vi "Sync clocks.vi"() -> ()   [LabVIEW 2019]
uses:
  <vilib>/Utility/error.llb/DialogType.ctl
  <vilib>/DAQmx/write.llb/DAQmx Write (Analog 2D DBL NChan NSamp).vi
  <vilib>/DAQmx/read.llb/DAQmx Read (Analog 2D DBL NChan NSamp).vi
  <vilib>/DAQmx/create/channels.llb/DAQmx Create Channel (AI-Voltage-Basic).vi
  <vilib>/DAQmx/configure/timing.llb/DAQmx Timing (Sample Clock).vi
  <vilib>/DAQmx/configure/trigger.llb/DAQmx Reference Trigger (Digital Edge).vi
  <vilib>/DAQmx/create/channels.llb/DAQmx Create Channel (AO-Voltage-Basic).vi
  <vilib>/DAQmx/configure/trigger.llb/DAQmx Start Trigger (Digital Edge).vi
  <vilib>/DAQmx/configure/trigger.llb/DAQmx Start Trigger (Time).vi
  <vilib>/DAQmx/configure/trigger.llb/DAQmx Start Trigger (Analog Edge).vi
  <vilib>/DAQmx/miscellaneous.llb/DAQmx Fill In Error Info.vi
  <resource>/objmgr/daqmx.rc
panel:
  out "standard output":string
  out "standard error":string
  out "return code":i32
  out "error out":errorcluster
  in  "command line":string
  in  "standard input":string
  in  "error in (no error)":errorcluster
  out "Execution Time (ms)":u32=13382
  out "Stop Tick":u32=2219165183
  out "Start Tick":u32=2219151801
  out "Acquired Samples":dbl[][](array[numeric]) format="%0.2f"
  out "Acquired Data":dbl[][](graph)
  out "Sampled Data Array Size":i32[](array[numeric])
  out "number of samples written per channel":u32
  out "binaryArraySize":i32[](array[numeric])
  in  "Transmit File Path":path=path "/media/sdc1/TempOATS1.bin"
  out "Current Acquired Data File":path=path "/media/sdc1/Temp220825212226.bin"
  in  "File Name Prefix":string="Temp"
  in  "path 2":path=path "/media/sdc1"
  out "free (bytes)":i64=2925575569408
  out "size (bytes)":i64=2999825367040
  out "folder names":string[](array[string])=["$RECYCLE.BIN", "29_Mar_noWind_Wave", "30_Mar_pier", "31_Mar_pier", "Bootcamp_recordings_SOARS", "IMTLab Wave Maker-12-21-21", "SOARS Software IMT Lab 032422", "System Volume Information", "TFOBootcamp2022_Day2", "TFO_Day3_signals", "TFO_Day4_signals", "temp"]
  out "filenames":string[](array[string])=[".dropbox.device", "Crack open SOARS binary log file 032422.vi", "IMTLab SOARS Datalogger.vi", "PolarPulldown_032422.bin", "Temp.bin", "Temp220407000420.bin", "Temp220825212058.bin", "Temp220825212226.bin"]
  in  "cDAQ Data File Path":path=path "/media/sdc1"
  in  "AI pretrigger samples per channel":u32=2
  in  "AI Trigger Edge":i32(ring)=10280 items=["Rising"=10280, "Falling"=10171]
  in  "AI Trigger Source":tag="/cDAQ1/ao/SampleClock"
  out "AI SampClk.Rate":dbl
  in  "AI Clock Source":tag="OnboardClock"
  in  "physical channels":tag="cDAQ1Mod1/ai0:3"
  in  "Trigger Type":T1(tab)
  in  "Digital Start Trigger Edge":i32(ring)=10280 caption="Edge" items=["Rising"=10280, "Falling"=10171]
  in  "Digital Start Trigger Source":tag="/Dev1/PFI0" caption="Source"
  in  "Digital Pause Trigger Pause When":i32(ring)=10192 caption="Pause When" items=["High"=10192, "Low"=10214]
  in  "Digital Pause Trigger Source":tag="/Dev1/PFI0" caption="Source"
  in  "Analog Start Trigger Level":dbl caption="Level" format="%0.2f"
  in  "Analog Start Trigger Hysteresis":dbl caption="Hysteresis" format="%.2f"
  in  "Analog Start Trigger Slope":i32(ring)=10280 caption="Slope" items=["Rising"=10280, "Falling"=10171]
  in  "Analog Start Trigger Source":string="APFI0" caption="Source"
  in  "Analog Pause Trigger Source":string="APFI0" caption="Source"
  in  "Analog Pause Trigger Pause When":i32(ring)=10093 caption="Pause When" items=["Above Level"=10093, "Below Level"=10107]
  in  "Analog Pause Trigger Level":dbl caption="Level" format="%.2f"
  in  "When":timestamp
  in  "Select Time\nManually":bool
  out "Data to Transmit":dbl[][](graph)
  out "Number of Samples":i32
  in  "Sample Rate":dbl=1000000.0
  in  "AO Sample Clock Source":tag="OnboardClock"
  in  "Max Voltage":dbl=5.0
  in  "Min Voltage":dbl=-5.0
  in  "Physical Channel(s)":tag="cDAQ1Mod2/ao0:3"
  out "Actual Sample Rate":dbl format="%0.2f"
  # "To enable triggers, select a tab above, and configure the settings.\n\nNot all hardware supports all trigger types. Refer to your device documentation for more information."
  # "This trigger type is not supported in output tasks. \n\nRefer to your device documentation for more information on which triggers are supported."
  # "This trigger type is not supported in output tasks. \n\nRefer to your device documentation for more information on which triggers are supported."
  # "If time is not manually set, task will begin after 10 seconds"
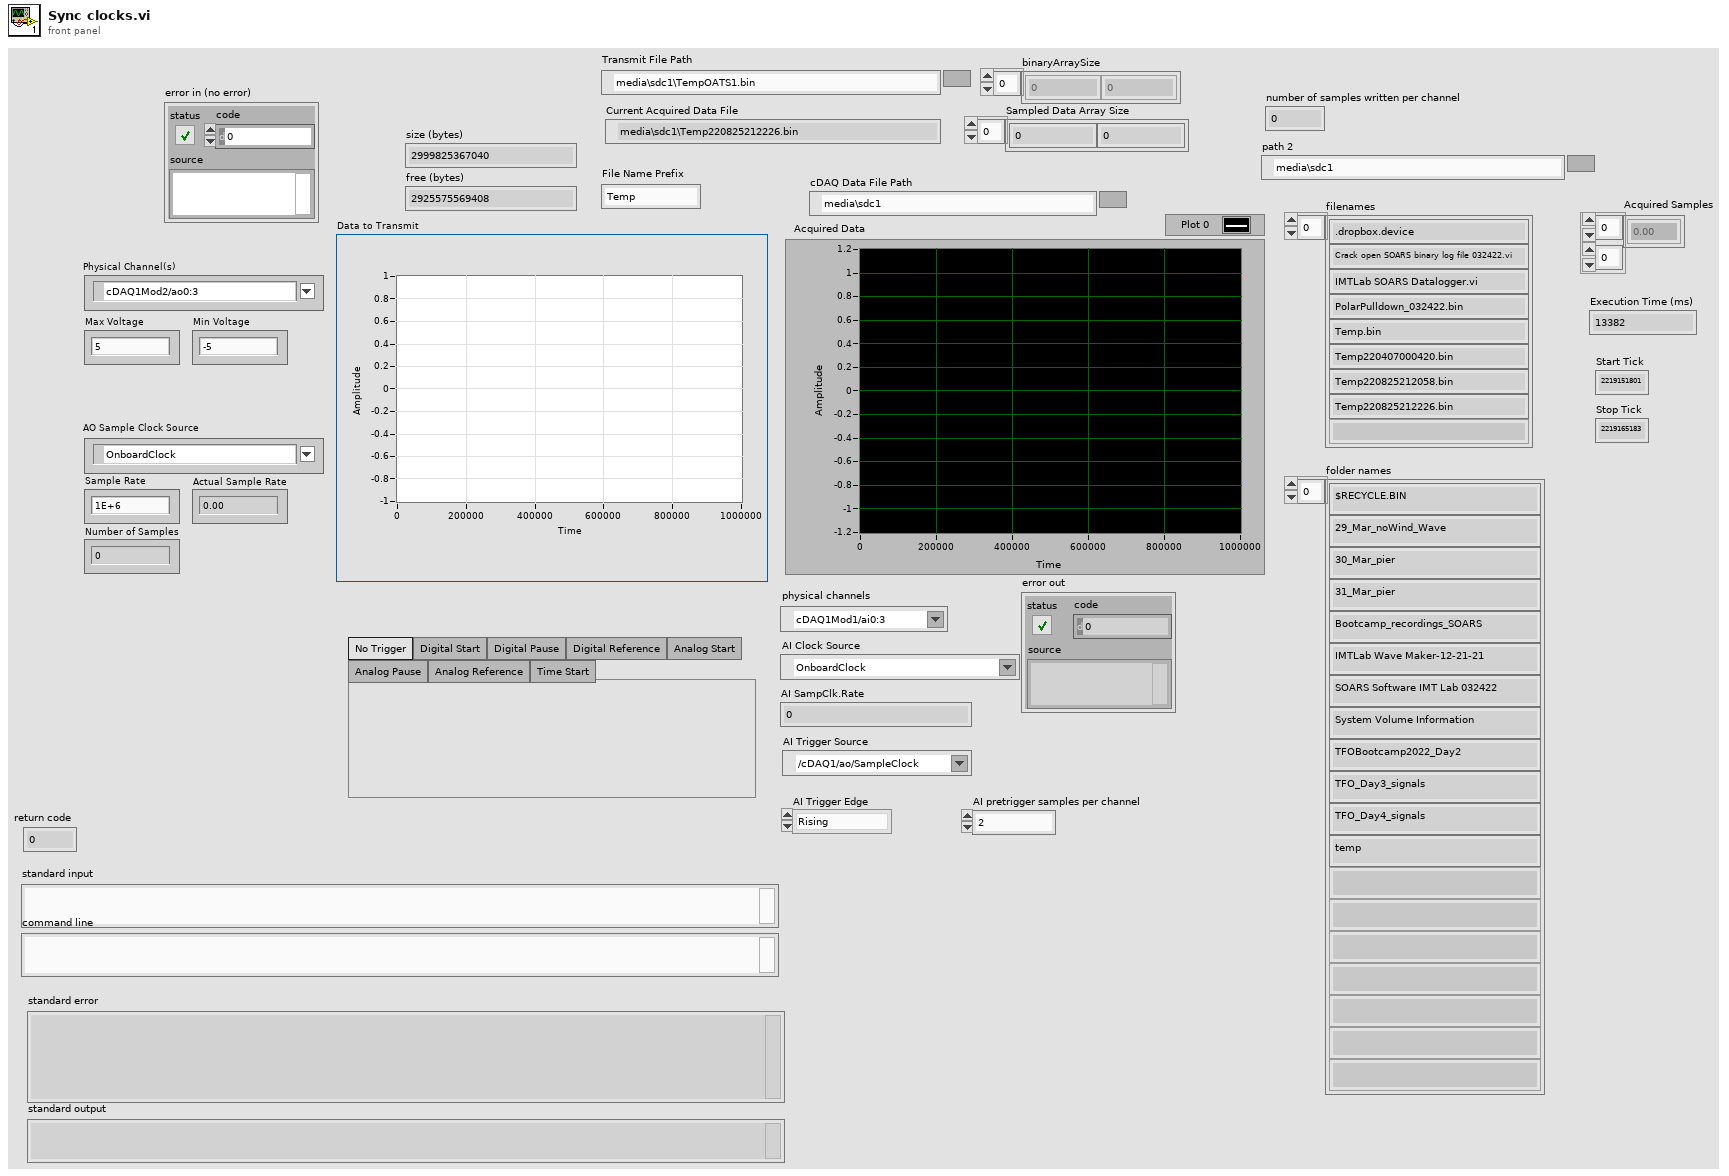
[diagram p1: front panel]
types:
  T1 = enum32{"No Trigger", "Digital Start", "Digital Pause", "Digital Reference", "Analog Start", "Analog Pause", "Analog Reference", "Time Start"}
  T2 = enum16{"open", "replace", "create", "open or create", "replace or create", "replace or create with confirmation"}
  T3 = enum16{"big-endian, network order", "native, host order", "little-endian"}
  T4 = typedef "DialogType.ctl" = u16
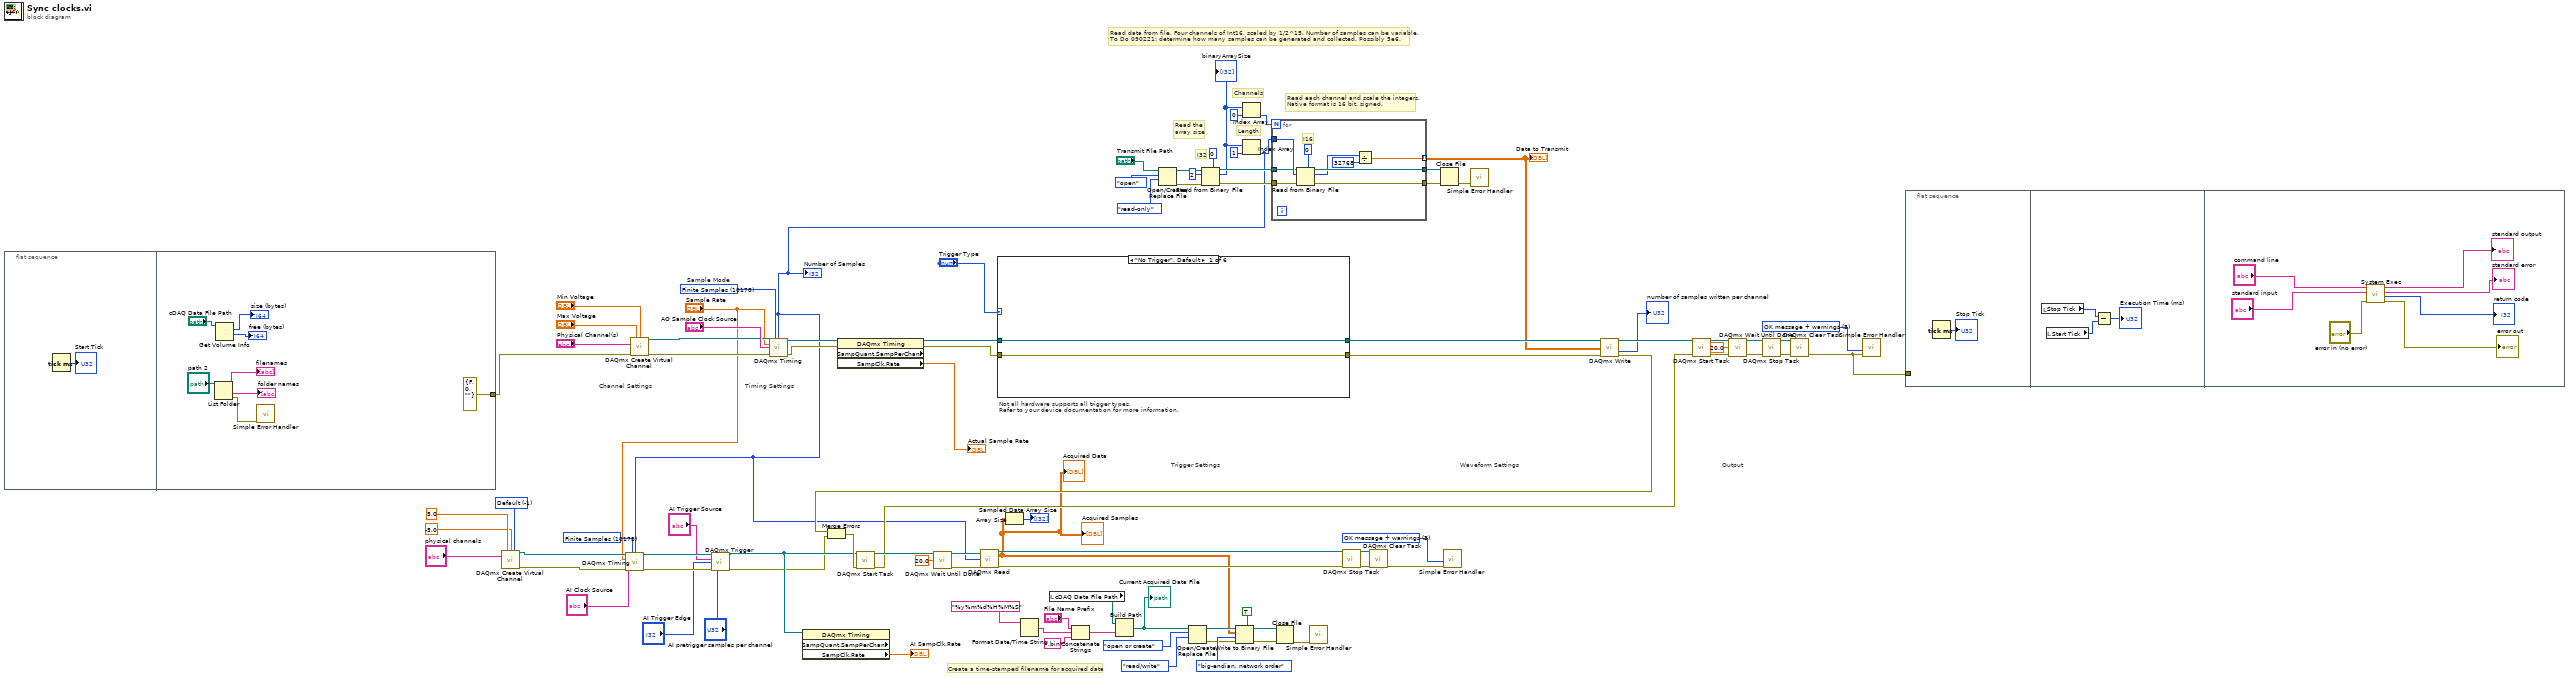
[diagram p0: block diagram]
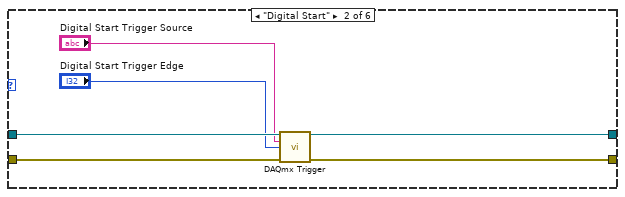
[diagram p2: hidden frame]
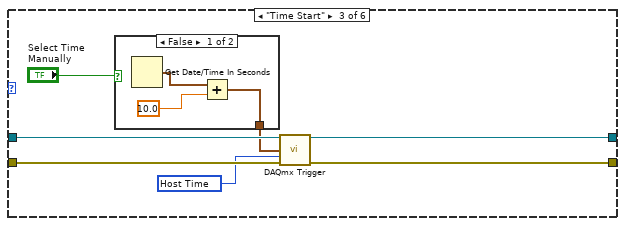
[diagram p3: hidden frame]
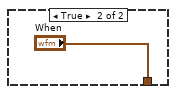
[diagram p4: hidden frame]
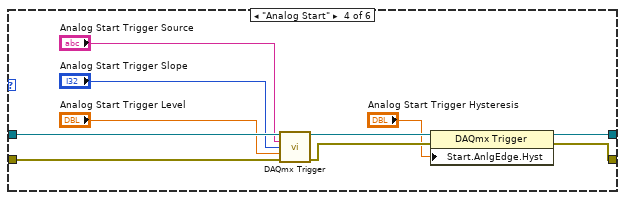
[diagram p5: hidden frame]
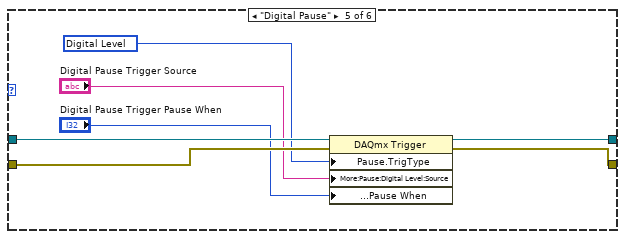
[diagram p6: hidden frame]
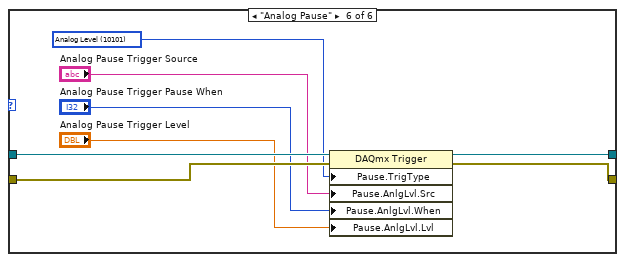
[diagram p7: hidden frame]
diagram:
  w57 = 10178 items=["Finite Samples"=10178, "Continuous Samples"=10123, "Hardware Timed Single Point"=12522] ("sample mode")
  w64 = T4 3 items=["no dialog", "OK message", "continue or stop message", "OK message + warnings", "continue/stop + warnings"] ("type of dialog (OK msg:1)")
  w69 = -1 items=["Default"=-1, "RSE"=10083, "NRSE"=10078, "Differential"=10106, "Pseudodifferential"=12529] ("input terminal configuration")
  w78 = T4 3 items=["no dialog", "OK message", "continue or stop message", "OK message + warnings", "continue/stop + warnings"] ("type of dialog (OK msg:1)")
  w91 = 10178 items=["Finite Samples"=10178, "Continuous Samples"=10123, "Hardware Timed Single Point"=12522]  # Sample Mode
  # "Create a time-stamped filename for acquired data"
  # "Read each channel and scale the integers.\nNative format is 16 bit, signed."
  # "Length"
  # "Channels"
  # "Read the \narray size"
  # "Read data from file. Four channels of Int16, scaled by 1/2^15. Number of samples can be variable. \nTo Do 090221: determine how many samples can be generated and collected. Possibly 5e6."
  # "I32"
  # "Trigger Settings"
  # "Not all hardware supports all trigger types.\nRefer to your device documentation for more information."
  # "Output"
  # "Waveform Settings"
  # "Timing Settings"
  # "Channel Settings"
  n1 = flat-sequence {
    tunnel: [errorcluster {"status"=FALSE, "code"=0, "source"=""} ("error constant")] -> w41
    frame #0 {
      n2 = Tick Count (ms)() -> (millisecond timer value=→"Start Tick":u32)
    }
    frame #1 {
      n3 = List Folder(path="path 2") -> (filenames=→"filenames":string[], folder names=→"folder names":string[], error out=w97:errorcluster)  [unwired: 3 in, 1 out]
      n4 = Get Volume Info(11:"cDAQ Data File Path") -> (1:→"free (bytes)":i64, 2:→"size (bytes)":i64)  [unwired: 1 in, 4 out]
      n5 = call <vilib>:"Simple Error Handler.vi"("error in (no error)"=w97) -> ()  [unwired: 4 in, 5 out]
    }
  }
  n6 = call-poly <vilib>:"DAQmx Create Virtual Channel.vi"("maximum value"=5.0, "minimum value"=-5.0, "input terminal configuration"=w69, "physical channels"="physical channels") -> ("task out"=w63:refnum<k21>, "error out"=w60:errorcluster)  [unwired: 10 in]
  n7 = call-poly <vilib>:"DAQmx Create Virtual Channel.vi"("maximum value"="Max Voltage", "minimum value"="Min Voltage", "physical channels"="Physical Channel(s)", "error in"=w41) -> ("task out"=w73:refnum<k21>, "error out"=w90:errorcluster)  [unwired: 10 in]
  n8 = Format Date/Time String(time format string (%c)="%y%m%d%H%M%S") -> (date/time string=w37:string)  [unwired: 2 in]
  n9 = local read "cDAQ Data File Path"() -> (w40:path)
  n10 = Concatenate Strings("File Name Prefix", w37, ".bin" ("string")) -> (w35:string)
  n11 = Build Path(base path=w40, name or relative path=w35) -> (appended path=w34:path)
  "Current Acquired Data File" <- w34
  n12 = Open/Create/Replace File(file path (use dialog)="Transmit File Path", operation (0:open)=T2."open", access (0:read/write)=enum16{"read/write", "read-only", "write-only"}."read-only") -> (refnum out=w22:refnum<file>, error out=w21:errorcluster)  [unwired: 3 in, 1 out]
  n13 = Open/Create/Replace File(file path (use dialog)=w34, operation (0:open)=T2."open or create", access (0:read/write)=enum16{"read/write", "read-only", "write-only"}."read/write") -> (refnum out=w31:refnum<file>, error out=w29:errorcluster)  [unwired: 3 in, 1 out]
  n14 = Read from Binary File(5:0, 8:w21, 10:2 ("count (1)"), 11:w22) -> (0:w15:errorcluster, 2:w8:i32[], 3:w13:refnum<file>)  [unwired: 2 in, 1 out]
  "binaryArraySize" <- w8
  n15 = Index Array(array=w8, index=0) -> (element=w17:i32)
  n16 = Index Array(array=w8, index=1) -> (element=w3:i32)
  "Number of Samples" <- w3
  n17 = call-poly <vilib>:"DAQmx Timing.vi"("task/channels in"=w63, "sample mode"=w57, "samples per channel"=w3, "rate"="Sample Rate", "source"="AI Clock Source", "error in"=w60) -> ("task out"=w50:refnum<k21>, "error out"=w48:errorcluster)  [unwired: 8 in]
  n18 = call-poly <vilib>:"DAQmx Trigger.vi"("task/channels in"=w50, "source"="AI Trigger Source", "edge"="AI Trigger Edge", "error in"=w48, "pretrigger samples per channel"="AI pretrigger samples per channel") -> ("task out"=w49:refnum<k21>, "error out"=w47:errorcluster)  [unwired: 9 in]
  n19 = call-poly <vilib>:"DAQmx Timing.vi"("task/channels in"=w73, "sample mode"=w91, "samples per channel"=w3, "rate"="Sample Rate", "source"="AO Sample Clock Source", "error in"=w90) -> ("task out"=w93:refnum<k21>, "error out"=w92:errorcluster)  [unwired: 8 in]
  n20 = property class="DAQmx Timing" props=["SampQuant.SampPerChan", "SampClk.Rate"](reference=w49) -> ("SampClk.Rate"=→"AI SampClk.Rate":dbl)  [unwired: 1 in, 3 out]
  n21 = property class="DAQmx Timing" props=["SampQuant.SampPerChan", "SampClk.Rate"](reference=w93, error in=w92) -> (reference out=w74:refnum<k21>, error out=w75:errorcluster, "SampClk.Rate"=→"Actual Sample Rate":dbl)  [unwired: 1 out]
  n22 = case shown="\"No Trigger\", Default" "Trigger Type" {
    tunnel: w74 -> [w104 w110 w117 w131 w138 w146]
    tunnel: w75 -> [w103 w109 w116 w130 w135 w143]
    tunnel: [w104 w108 w115 w128 w137 w145] -> w76
    tunnel: [w103 w107 w114 w127 w136 w144] -> w24
    frame "No Trigger", Default {
    }
    frame "Digital Start" {
      n23 = call-poly <vilib>:"DAQmx Trigger.vi"("task/channels in"=w110, "source"="Digital Start Trigger Source", "edge"="Digital Start Trigger Edge", "error in"=w109) -> ("task out"=w108:refnum<k21>, "error out"=w107:errorcluster)  [unwired: 10 in]
    }
    frame "Time Start" {
      w113 = 16126 items=["Host Time"=16126, "I/O Device Time"=16127] ("timescale")
      n24 = case shown="False" "Select Time\nManually" {
        tunnel: [w119 "When"] -> w111
        frame False {
          n25 = Get Date/Time In Seconds() -> (seconds since 1Jan1904=w120:timestamp)
          n26 = Add(x=w120, y=10.0) -> (x+y=w119:timestamp)
        }
        frame True {
        }
      }
      n27 = call-poly <vilib>:"DAQmx Trigger.vi"("task/channels in"=w117, "when"=w111, "timescale"=w113, "error in"=w116) -> ("task out"=w115:refnum<k21>, "error out"=w114:errorcluster)  [unwired: 10 in]
    }
    frame "Analog Start" {
      n28 = call-poly <vilib>:"DAQmx Trigger.vi"("task/channels in"=w131, "source"="Analog Start Trigger Source", "slope"="Analog Start Trigger Slope", "level"="Analog Start Trigger Level", "error in"=w130) -> ("task out"=w126:refnum<k21>, "error out"=w125:errorcluster)  [unwired: 9 in]
      n29 = property class="DAQmx Trigger"(reference=w126, error in=w125, "Start.AnlgEdge.Hyst"="Analog Start Trigger Hysteresis") -> (reference out=w128:refnum<k21>, error out=w127:errorcluster)
    }
    frame "Digital Pause" {
      w134 = 10152 items=["Analog Level"=10101, "Analog Window"=10103, "Digital Level"=10152, "Digital Pattern"=10398, "None"=10230] ("Pause.TrigType")
      n30 = property class="DAQmx Trigger"(reference=w138, error in=w135, "Pause.TrigType"=w134, "More:Pause:Digital Level:Source"="Digital Pause Trigger Source", "More:Pause:Digital Level:Pause When"="Digital Pause Trigger Pause When") -> (reference out=w137:refnum<k21>, error out=w136:errorcluster)
    }
    frame "Analog Pause" {
      w142 = 10101 items=["Analog Level"=10101, "Analog Window"=10103, "Digital Level"=10152, "Digital Pattern"=10398, "None"=10230] ("Pause.TrigType")
      n31 = property class="DAQmx Trigger"(reference=w146, error in=w143, "Pause.TrigType"=w142, "Pause.AnlgLvl.Src"="Analog Pause Trigger Source", "Pause.AnlgLvl.When"="Analog Pause Trigger Pause When", "Pause.AnlgLvl.Lvl"="Analog Pause Trigger Level") -> (reference out=w145:refnum<k21>, error out=w144:errorcluster)
    }
  }
  n32 = for {
    N: w17 -> [_]
    tunnel: w3 -> [w155]
    tunnel: w15 -> [w153]
    tunnel: [w152] -> w14
    tunnel: w13 -> [w151]
    tunnel: [w150] -> w12
    tunnel: [w147] -> w9 mode=indexing
    # "I16"
    n33 = Read from Binary File(5:i16 0, 8:w153, 10:w155, 11:w151) -> (0:w152:errorcluster, 2:w149:i16[], 3:w150:refnum<file>)  [unwired: 2 in, 1 out]
    n34 = Divide(x=w149, y=32768) -> (x/y=w147:dbl[])
  }
  "Data to Transmit" <- w9
  n35 = Close File(refnum=w12, error in=w14) -> (error out=w2:errorcluster)  [unwired: 1 out]
  n36 = call <vilib>:"Simple Error Handler.vi"("error in (no error)"=w2) -> ()  [unwired: 4 in, 5 out]
  n37 = call-poly <vilib>:"DAQmx Write.vi"("task/channels in"=w76, "data"=w9, "error in"=w24) -> ("task out"=w85:refnum<k21>, "number of samples written per channel"=→"number of samples written per channel":u32, "error out"=w56:errorcluster)  [unwired: 10 in]
  n38 = Merge Errors(w56, w47) -> (w55:errorcluster)
  n39 = call <vilib>:"DAQmx Start Task.vi"("task/channels in"=w49, "error in"=w55) -> ("task out"=w67:refnum<k21>, "error out"=w54:errorcluster)  [unwired: 12 in]
  n40 = call <vilib>:"DAQmx Wait Until Done.vi"("task/channels in"=w67, "timeout (sec)"=20.0) -> ("task out"=w62:refnum<k21>, "error out"=w59:errorcluster)  [unwired: 12 in]
  n41 = call-poly <vilib>:"DAQmx Read.vi"("task/channels in"=w62, "number of samples per channel"=w3, "error in"=w59) -> ("task out"=w61:refnum<k21>, "data"=w4:dbl[][], "error out"=w58:errorcluster)  [unwired: 10 in]
  "Acquired Data" <- w4
  "Acquired Samples" <- w4
  n42 = Array Size(array=w4) -> (size(s)=→"Sampled Data Array Size":i32[])
  n43 = Write to Binary File(file (use dialog)=w31, data=w4, error in=w29, 5:TRUE ("prepend array or string size? (T)"), 9:T3."big-endian, network order" ("byte order (0:big-endian, network order)")) -> (refnum out=w26:refnum<file>, error out=w27:errorcluster)  [unwired: 1 in, 1 out]
  n44 = Close File(refnum=w26, error in=w27) -> (error out=w25:errorcluster)  [unwired: 1 out]
  n45 = call <vilib>:"Simple Error Handler.vi"("error in (no error)"=w25) -> ()  [unwired: 4 in, 5 out]
  n46 = call <vilib>:"DAQmx Stop Task.vi"("task/channels in"=w61, "error in"=w58) -> ("task out"=w66:refnum<k21>, "error out"=w65:errorcluster)  [unwired: 12 in]
  n47 = call <vilib>:"DAQmx Clear Task.vi"("task in"=w66, "error in"=w65) -> ("error out"=w68:errorcluster)  [unwired: 13 in]
  n48 = call <vilib>:"Simple Error Handler.vi"("type of dialog (OK msg:1)"=w64, "error in (no error)"=w68) -> ()  [unwired: 3 in, 5 out]
  n49 = call <vilib>:"DAQmx Start Task.vi"("task/channels in"=w85, "error in"=w54) -> ("task out"=w84:refnum<k21>, "error out"=w83:errorcluster)  [unwired: 12 in]
  n50 = call <vilib>:"DAQmx Wait Until Done.vi"("task/channels in"=w84, "timeout (sec)"=20.0, "error in"=w83) -> ("task out"=w80:refnum<k21>, "error out"=w79:errorcluster)  [unwired: 11 in]
  n51 = call <vilib>:"DAQmx Stop Task.vi"("task/channels in"=w80, "error in"=w79) -> ("task out"=w82:refnum<k21>, "error out"=w81:errorcluster)  [unwired: 12 in]
  n52 = call <vilib>:"DAQmx Clear Task.vi"("task in"=w82, "error in"=w81) -> ("error out"=w1:errorcluster)  [unwired: 13 in]
  n53 = call <vilib>:"Simple Error Handler.vi"("type of dialog (OK msg:1)"=w78, "error in (no error)"=w1) -> ()  [unwired: 3 in, 5 out]
  n54 = flat-sequence {
    tunnel: w1 -> [_]
    frame #0 {
      n55 = Tick Count (ms)() -> (millisecond timer value=→"Stop Tick":u32)
    }
    frame #1 {
      n56 = local read "Stop Tick"() -> (w159:u32)
      n57 = local read "Start Tick"() -> (w158:u32)
      n58 = Subtract(x=w159, y=w158) -> (x-y=→"Execution Time (ms)":u32)
    }
    frame #2 {
      n59 = call <vilib>:"System Exec.vi"("error in (no error)"="error in (no error)", "standard input"="standard input", "command line"="command line") -> ("error out"=→"error out":errorcluster, "return code"=→"return code":i32, "standard error"=→"standard error":string, "standard output"=→"standard output":string)  [unwired: 5 in]
    }
  }
